vi "Reporting_proc_energia_inycom.vi"(1 "Datos":dbl[][](array[numeric])) -> (0 "String":string)   [LabVIEW 2015]
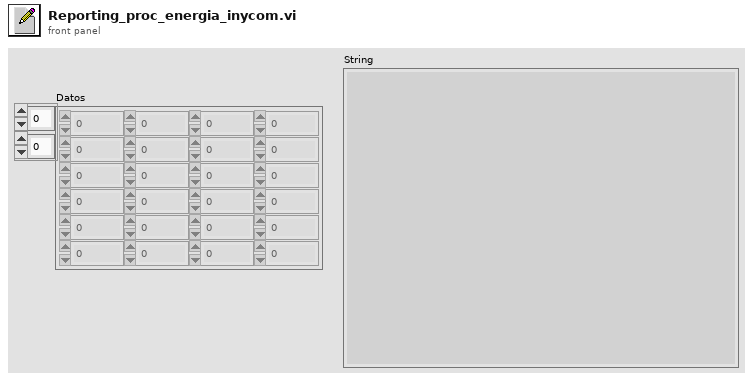
[diagram p1: front panel]
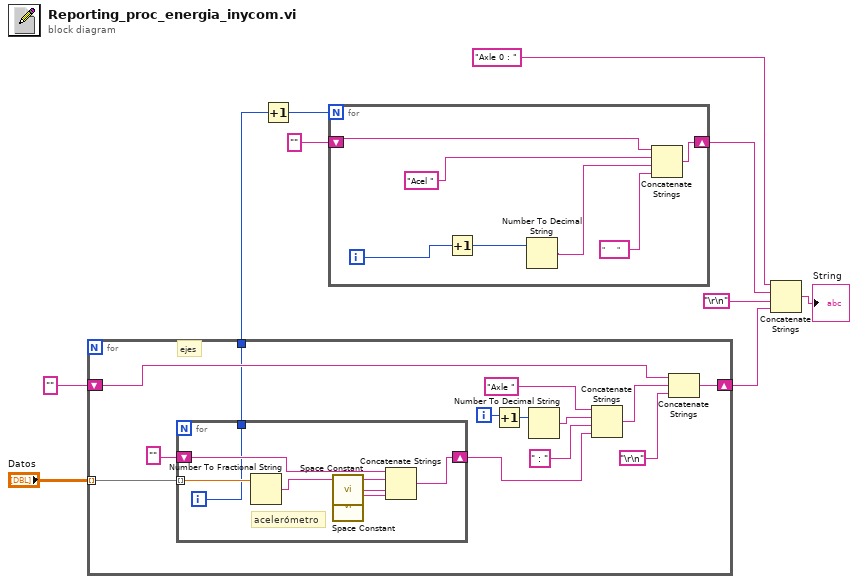
[diagram p0: block diagram]
diagram:
  n1 = for {
    tunnel: "Datos" -> [w23] mode=indexing
    shift-right: [w22] -> w4
    shift-left: "" -> [w21]
    tunnel: [w12] -> w1
    i -> [w18]
    # "ejes"
    n2 = for {
      tunnel: w23 -> [w30] mode=indexing
      shift-right: [w26] -> w14
      shift-left: "" -> [w25]
      tunnel: [w24] -> w12
      i -> [w24]
      # "acelerómetro"
      n3 = Number To Fractional String(number=w30) -> (F-format string=w29:string)  [unwired: 3 in]
      n4 = call <vilib>:"Space Constant.vi"() -> ("String"=w28:string)
      n5 = call <vilib>:"Space Constant.vi"() -> ("String"=w27:string)
      n6 = Concatenate Strings(w25, w29, w28, w27) -> (w26:string)
    }
    n7 = Increment(x=w18) -> (x+1=w17:i32)
    n8 = Number To Decimal String(number=w17) -> (decimal integer string=w16:string)  [unwired: 1 in]
    n9 = Concatenate Strings("Axle " ("string"), w16, " : " ("string"), w14) -> (w13:string)
    n10 = Concatenate Strings(w21, w13, "\r\n") -> (w22:string)
  }
  n11 = Increment(x=w1) -> (x+1=w2:i32)
  n12 = for {
    N: w2 -> [_]
    shift-right: [w36] -> w6
    shift-left: "" -> [w35]
    i -> [w33]
    n13 = Increment(x=w33) -> (x+1=w32:i32)
    n14 = Number To Decimal String(number=w32) -> (decimal integer string=w31:string)  [unwired: 1 in]
    n15 = Concatenate Strings(w35, "Acel " ("string"), w31, "      " ("string")) -> (w36:string)
  }
  n16 = Concatenate Strings("Axle 0 : " ("string"), w6, "\r\n", w4) -> (→"String":string)
